vi "DO Dynamic Data Update.vi"(8 "error in":errorcluster, 11 "DO Config Data":T1) -> (0 "error out":errorcluster, 2 "Data to Generate":bool[](array[boolean]), 3 "DO Config Data 2":T1)   [LabVIEW 2024]
doc: "All Rights Reserved © 2017 SyncSols"
uses:
  Host-DQMH/Configuration/DO Channel's.ctl
  Host-DQMH/Configuration/Configuration.lvlib
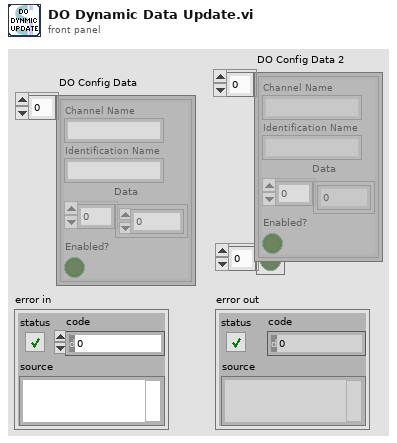
[diagram p1: front panel]
types:
  T1 = typedef "Configuration.lvlib/DO Channel's.ctl" = cluster{"Channel Name":string, "Identification Name":string, "Data":u8[], "Enabled?":bool}[]
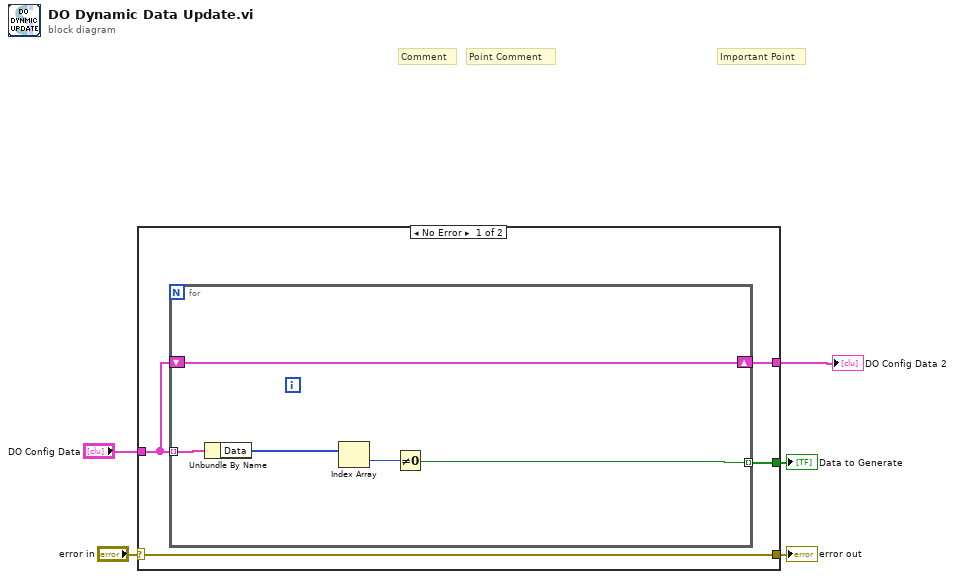
[diagram p0: block diagram]
diagram:
  # "Important Point"
  # "Point Comment"
  # "Comment"
  n1 = case shown="No Error" "error in" {
    selector: "error in" -> [w9 w16]
    tunnel: [w9 w16] -> w5
    tunnel: "DO Config Data" -> [w8 w15]
    tunnel: [w7 _] -> w3
    tunnel: [w6 w15] -> w2
    frame No Error {
      n2 = for {
        tunnel: w8 -> [w14] mode=indexing
        tunnel: [w12] -> w7 mode=indexing
        shift-right: [w11] -> w6
        shift-left: w8 -> [w11]
        n3 = Unbundle By Name(w14) -> ("Data"=w13:u8[])
        n4 = Index Array(array=w13) -> (element=w10:u8)  [unwired: 1 in]
        n5 = Not Equal To 0?(x=w10) -> (x != 0?=w12:bool)
      }
    }
    frame Error {
    }
  }
  "error out" <- w5
  "Data to Generate" <- w3
  "DO Config Data 2" <- w2
